vi "Supported Music Libraries Plugins Path.vi"() -> (5 "Supported Music Libraries Plugins Path":path)   [LabVIEW 2015, in "App Config.lvlib"]
uses:
  App Config.lvlib
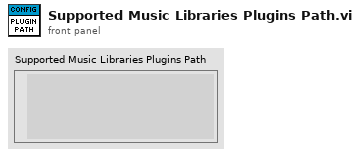
[diagram p1: front panel]
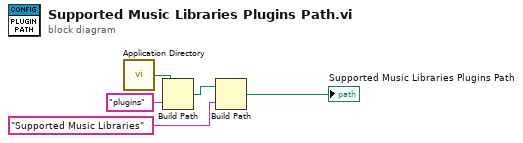
[diagram p0: block diagram]
diagram:
  n1 = call <vilib>:"Application Directory.vi"() -> ("Application Directory"=w4:path)
  n2 = Build Path(base path=w4, name or relative path="plugins") -> (appended path=w3:path)
  n3 = Build Path(base path=w3, name or relative path="Supported Music Libraries") -> (appended path=→"Supported Music Libraries Plugins Path":path)
